vi "trigger_holdoff.vi"(7 "error in (no error)":errorcluster {"code" format="%.0x"}, 9 "Holdoff Time":dbl, 10 "VISA Scope In":refnum<visa-resource-name>) -> (0 "error out":errorcluster {"code" format="%.0x"}, 3 "VISA Out":refnum<visa-resource-name>)   [LabVIEW 2011]
panel:
  out "Sent String":string
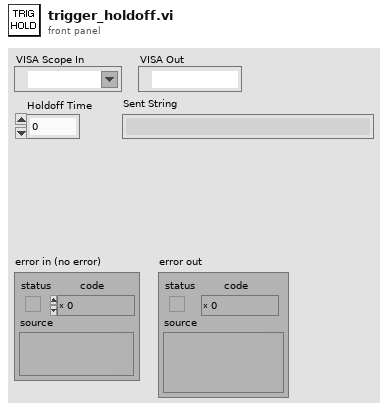
[diagram p1: front panel]
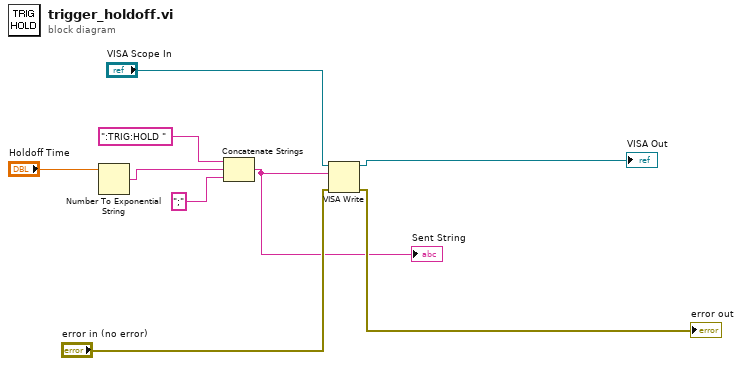
[diagram p0: block diagram]
diagram:
  n1 = Number To Exponential String(number="Holdoff Time") -> (E-format string=w7:string)  [unwired: 3 in]
  n2 = Concatenate Strings(":TRIG:HOLD " ("string"), w7, ";" ("string")) -> (w1:string)
  "Sent String" <- w1
  n3 = VISA Write(VISA resource name="VISA Scope In", write buffer=w1, error in (no error)="error in (no error)") -> (VISA resource name out=→"VISA Out":refnum<visa-resource-name>, error out=→"error out":errorcluster)  [unwired: 1 out]
